vi "Variant to Type.vi"(11 "Value":variant) -> (3 "Value Type":T1)   [LabVIEW 2020, in "Parallel Block.lvlib"]
uses:
  Parallel Block.lvlib
  <vilib>/Utility/Data Type/NI_Data Type.lvlib
  <vilib>/IlluminatedG/lv-stream/Stream.lvlib
  Value Type.ctl
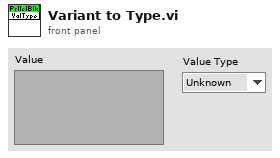
[diagram p1: front panel]
types:
  T1 = typedef "Parallel Block.lvlib/Value Type.ctl" = enum16{"Unknown", "Bool", "U8", "U16", "U32", "U64", "I8", "I16", "I32", "I64", "SGL", "DBL", "CSG", "CDB", "CDBWfm", "String", "DBLWfm"}
  T2 = typedef "NI_Data Type.lvlib/Data Type.ctl" = enum8{"Invalid Type", "Void", "I8", "I16", "I32", "I64", "U8", "U16", "U32", "U64", "Single Float", "Double Float", "Extended Float", "Single Complex", "Double Complex", "Extended Complex", "Enum U8", "Enum U16", "Enum U32", "Enum U64", "Single Float With Unit", "Double Float With Unit", "Extended Float With Unit", "Single Complex with Unit", "Double Complex with Unit", "Extended Complex with Unit", "Boolean", "String", "Path", "Picture", "Tag", "Array", "Cluster", "Variant", "LV Variant", "Waveform", "Timestamp", "Digital Waveform", "Digital Data", "ExpressData", "Refnum", "External Data", "VI", "Poly VI", "LabVIEW Class Instance", "Fixed Point", "Set Collection", "Map Collection"}
  T3 = typedef "NI_Data Type.lvlib/Type Definition Info.ctl" = cluster{"Name":string, "Timestamp":u32}
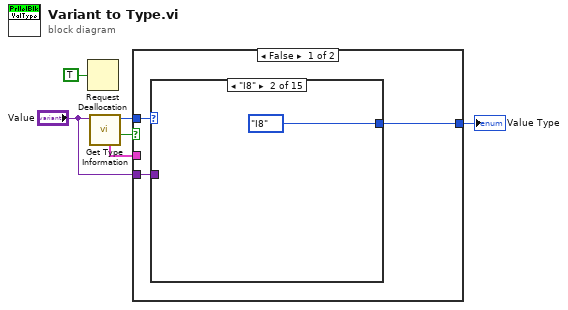
[diagram p0: block diagram]
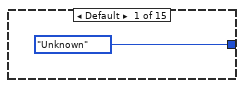
[diagram p2: hidden frame]
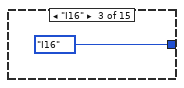
[diagram p3: hidden frame]
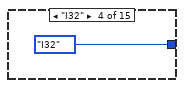
[diagram p4: hidden frame]
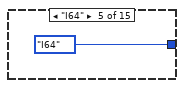
[diagram p5: hidden frame]
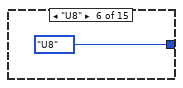
[diagram p6: hidden frame]
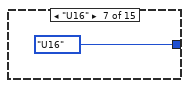
[diagram p7: hidden frame]
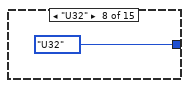
[diagram p8: hidden frame]
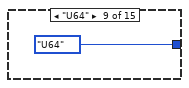
[diagram p9: hidden frame]
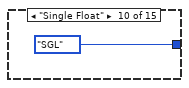
[diagram p10: hidden frame]
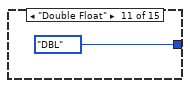
[diagram p11: hidden frame]
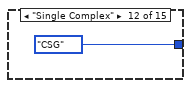
[diagram p12: hidden frame]
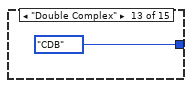
[diagram p13: hidden frame]
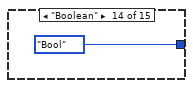
[diagram p14: hidden frame]
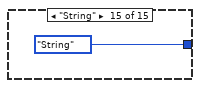
[diagram p15: hidden frame]
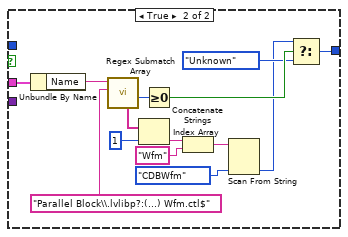
[diagram p16: hidden frame]
diagram:
  n1 = Request Deallocation(TRUE ("flag")) -> ()
  n2 = call <vilib>:"Get Type Information.vi"("variant"="Value") -> ("type definition"=w4:bool, "type"=w3:T2, "type definition info"=w5:T3)  [unwired: 6 in, 2 out]
  n3 = case shown="False" w4 {
    tunnel: w5 -> [_ w38]
    tunnel: w3 -> [w9 _]
    tunnel: [w8 w32] -> w2
    tunnel: "Value" -> [w7 _]
    frame False {
      n4 = case shown="\"I8\"" w9 {
        tunnel: [Value_Type."Unknown" ("Value Type") Value_Type."I8" ("Value Type") Value_Type."I16" ("Value Type") Value_Type."I32" ("Value Type") Value_Type."I64" ("Value Type") Value_Type."U8" ("Value Type") Value_Type."U16" ("Value Type") Value_Type."U32" ("Value Type") Value_Type."U64" ("Value Type") Value_Type."SGL" ("Value Type") Value_Type."DBL" ("Value Type") Value_Type."CSG" ("Value Type") Value_Type."CDB" ("Value Type") Value_Type."Bool" ("Value Type") Value_Type."String" ("Value Type")] -> w8
        tunnel: w7 -> [_ _ _ _ _ _ _ _ _ _ _ _ _ _ _]
        frame Default {
        }
        frame "I8" {
        }
        frame "I16" {
        }
        frame "I32" {
        }
        frame "I64" {
        }
        frame "U8" {
        }
        frame "U16" {
        }
        frame "U32" {
        }
        frame "U64" {
        }
        frame "Single Float" {
        }
        frame "Double Float" {
        }
        frame "Single Complex" {
        }
        frame "Double Complex" {
        }
        frame "Boolean" {
        }
        frame "String" {
        }
      }
    }
    frame True {
      n5 = Unbundle By Name(w38) -> ("Name"=w37:string)
      n6 = call <vilib>:"Regex Submatch Array.vi"("regular expression"="Parallel Block\\.lvlibp?:(...) Wfm.ctl$", "string"=w37) -> ("offset past match"=w35:i32, "matches"=w31:string[])  [unwired: 5 in, 3 out]
      n7 = Index Array(array=w31, index=1) -> (element=w29:string)
      n8 = Greater Or Equal To 0?(x=w35) -> (x >= 0?=w34:bool)
      n9 = Concatenate Strings(w29, "Wfm") -> (w27:string)
      n10 = Scan From String(input string=w27, default 1=Value_Type."CDBWfm" ("Value Type")) -> (output 1=w25:T1)  [unwired: 3 in, 3 out]
      n11 = Select(t=w25, s=w34, f=Value_Type."Unknown" ("Value Type")) -> (s? t:f=w32:T1)
    }
  }
  "Value Type" <- w2
